vi "Excel___Lockout and Close.vi"(0 "Excel Ref In":refnum<k7>, 5 "WorkbookS Ref In":refnum<k7>, 7 "Workbook Ref In":refnum<k7>, 9 "Sheets Ref In":refnum<k7>, 11 "Error In":errorcluster) -> (15 "Error Out":errorcluster)   [LabVIEW 2013]
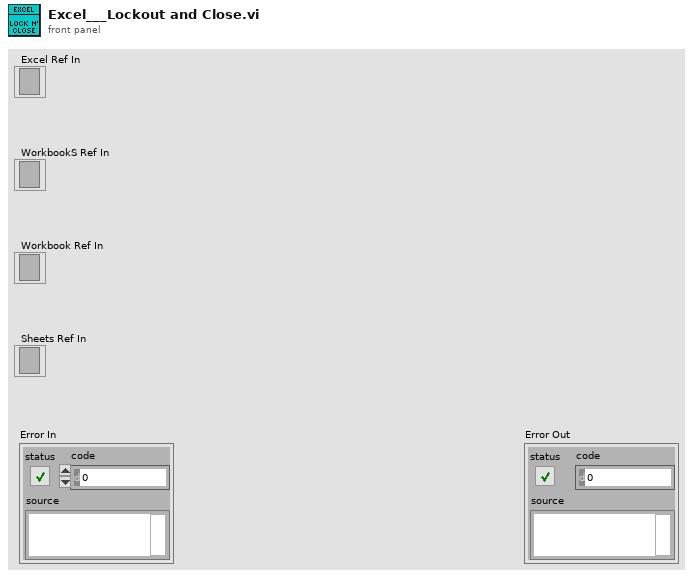
[diagram p1: front panel]
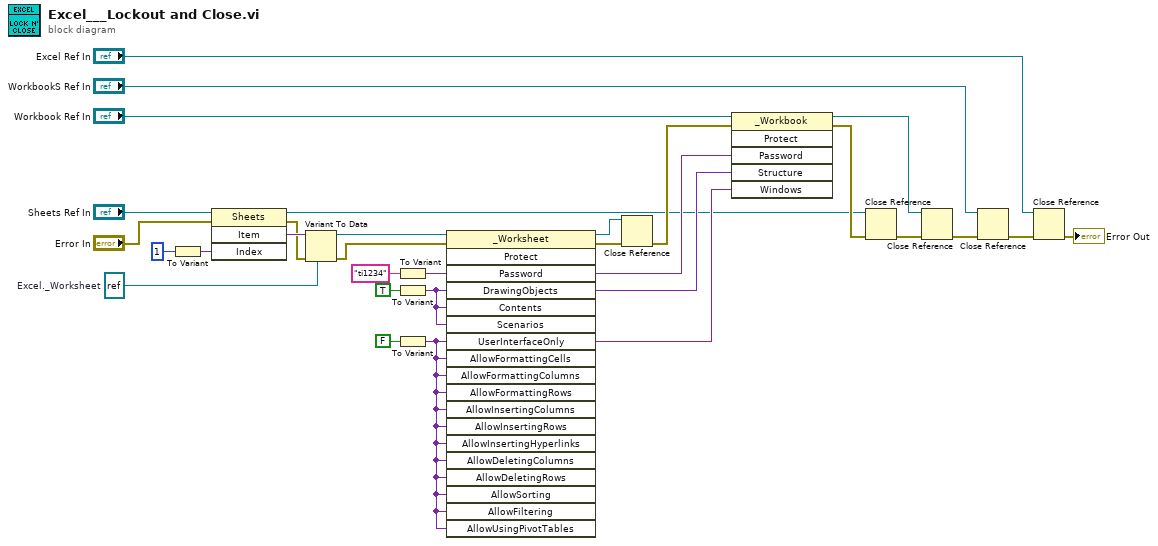
[diagram p0: block diagram]
diagram:
  w21 = refnum<k7> refnum  # Excel._Worksheet
  n1 = To Variant(anything=1) -> (Variant=w16:variant)
  n2 = invoke class="Sheets" method="Item"(reference="Sheets Ref In", error in="Error In", "Index"=w16) -> (reference out=w8:refnum<k7>, error out=w15:errorcluster, "Item"=w17:variant)  [unwired: 1 in, 1 out]
  n3 = Variant To Data(error in=w15, type=w21, Variant=w17) -> (data=w14:refnum<k7>, error out=w13:errorcluster)
  n4 = To Variant(anything="ti1234") -> (Variant=w26:variant)
  n5 = To Variant(anything=TRUE) -> (Variant=w27:variant)
  n6 = To Variant(anything=FALSE) -> (Variant=w28:variant)
  n7 = invoke class="_Worksheet" method="Protect"(reference=w14, error in=w13, "Password"=w26, "DrawingObjects"=w27, "Contents"=w27, "Scenarios"=w27, "UserInterfaceOnly"=w28, "AllowFormattingCells"=w28, "AllowFormattingColumns"=w28, "AllowFormattingRows"=w28, "AllowInsertingColumns"=w28, "AllowInsertingRows"=w28, "AllowInsertingHyperlinks"=w28, "AllowDeletingColumns"=w28, "AllowDeletingRows"=w28, "AllowSorting"=w28, "AllowFiltering"=w28, "AllowUsingPivotTables"=w28) -> (reference out=w12:refnum<k7>, error out=w11:errorcluster)  [unwired: 1 in, 17 out]
  n8 = Close Reference(reference=w12, error in (no error)=w11) -> (error out=w25:errorcluster)
  n9 = invoke class="_Workbook" method="Protect"(reference="Workbook Ref In", error in=w25, "Password"=w26, "Structure"=w27, "Windows"=w28) -> (reference out=w4:refnum<k7>, error out=w9:errorcluster)  [unwired: 1 in, 4 out]
  n10 = Close Reference(reference=w8, error in (no error)=w9) -> (error out=w7:errorcluster)
  n11 = Close Reference(reference=w4, error in (no error)=w7) -> (error out=w6:errorcluster)
  n12 = Close Reference(reference="WorkbookS Ref In", error in (no error)=w6) -> (error out=w5:errorcluster)
  n13 = Close Reference(reference="Excel Ref In", error in (no error)=w5) -> (error out=→"Error Out":errorcluster)
